vi "FTW-Test-Array-Shuffle.vi"() -> (0 "Test Result":errorcluster)   [LabVIEW 2015]
uses:
  src/error/FTW-ERR-ThrowInfo.vi
  src/error/FTW-ERR-ThrowError.vi
  src/error/FTW-ERR-CallChain.vi
  src/error/FTW-ERR-NoErrorConstant.vi
  src/string/FTW-STR-ReplaceWhitespace.vi
  src/string/FTW-STR-Array-Delimit.vi
  src/error/FTW-ERR-Clear.vi
  src/regex/FTW-Regex-ReplaceAll.vi
  codegen/xnode/FTW-Array-Shuffle.xnode
panel:
  out "Slope of Regression Line":dbl
  out "Differentials":dbl[](graph)
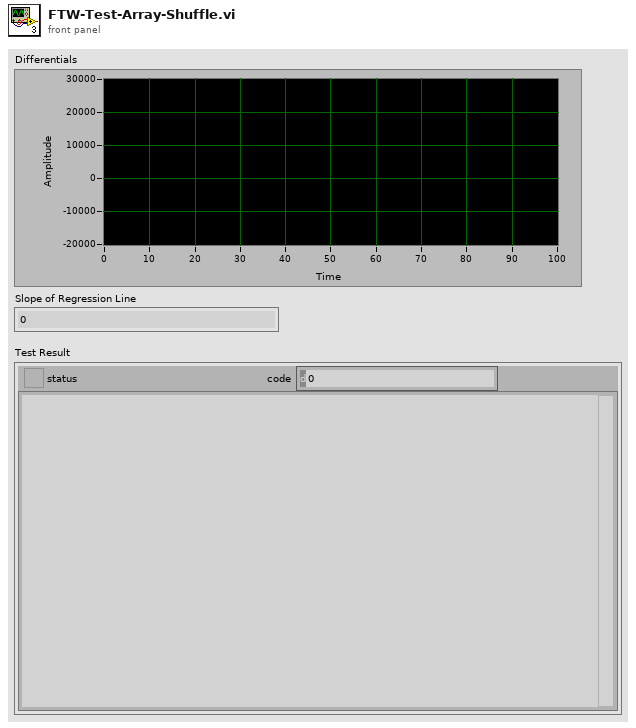
[diagram p1: front panel]
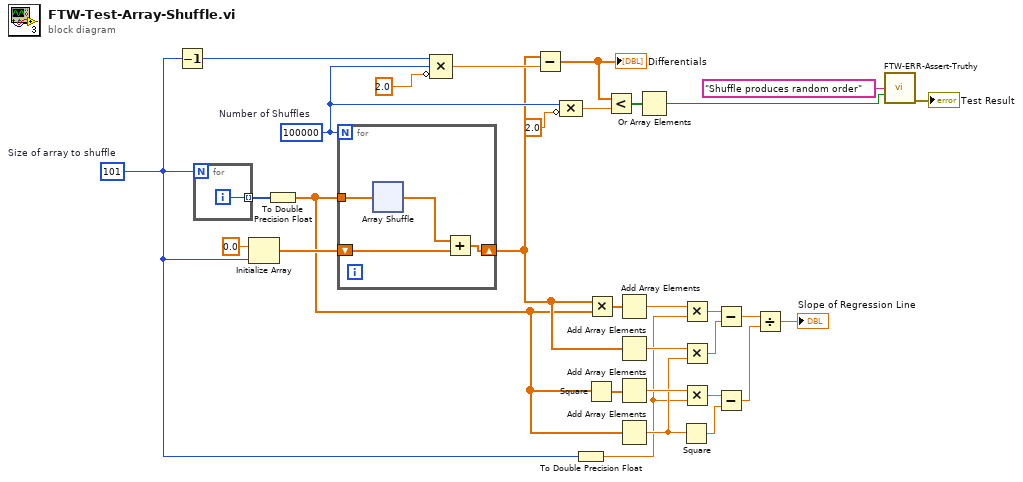
[diagram p0: block diagram]
diagram:
  w23 = 100000  # Number of Shuffles
  w11 = 101  # Size of array to shuffle
  n1 = Decrement(x=w11) -> (x-1=w28:i32)
  n2 = for {
    N: w11 -> [_]
    tunnel: [w32] -> w29 mode=indexing
    i -> [w32]
  }
  n3 = Initialize Array(0.0 ("element"), w11) -> (w30:dbl[])
  n4 = To Double Precision Float(number=w29) -> (double precision float=w14:dbl[])
  n5 = for {
    N: w23 -> [_]
    shift-right: [w34] -> w18
    shift-left: w30 -> [w35]
    tunnel: w14 -> [w33]
    n6 = xnode "Array Shuffle"("Array"=w33) -> ("Shuffled Array"=w36:dbl[])
    n7 = Add(x=w36, y=w35) -> (x+y=w34:dbl[])
  }
  n8 = Compound Arithmetic op=MULTIPLY(w28, w23, invert 2.0) -> (w26:dbl)
  n9 = Subtract(x=w18, y=w26) -> (x-y=w25:dbl[])
  "Differentials" <- w25
  n10 = Compound Arithmetic op=MULTIPLY(w23, invert 2.0) -> (w22:dbl)
  n11 = To Double Precision Float(number=w11) -> (double precision float=w4:dbl)
  n12 = Square(x=w14) -> (x^2=w13:dbl[])
  n13 = Multiply(x=w18, y=w14) -> (x*y=w20:dbl[])
  n14 = Less?(x=w25, y=w22) -> (x < y?=w24:bool[])
  n15 = Add Array Elements(numeric array=w20) -> (sum=w19:dbl)
  n16 = Add Array Elements(numeric array=w18) -> (sum=w17:dbl)
  n17 = Add Array Elements(numeric array=w13) -> (sum=w12:dbl)
  n18 = Add Array Elements(numeric array=w14) -> (sum=w9:dbl)
  n19 = Or Array Elements(Boolean array=w24) -> (logical OR=w3:bool)
  n20 = Square(x=w9) -> (x^2=w8:dbl)
  n21 = Multiply(x=w19, y=w4) -> (x*y=w16:dbl)
  n22 = Multiply(x=w17, y=w9) -> (x*y=w15:dbl)
  n23 = Multiply(x=w12, y=w4) -> (x*y=w7:dbl)
  n24 = Subtract(x=w16, y=w15) -> (x-y=w10:dbl)
  n25 = Subtract(x=w7, y=w8) -> (x-y=w6:dbl)
  n26 = Divide(x=w10, y=w6) -> (x/y=→"Slope of Regression Line":dbl)
  n27 = call "FTW-ERR-Assert-Truthy.vi"("Assertion"="Shuffle produces random order" ("Error Message"), "Assertion holds true?"=w3) -> ("error out"=→"Test Result":errorcluster)  [unwired: 13 in]
